vi "Set Clip Plane (no reference).vi"(8 "error in (no error)":errorcluster, 9 "Clip Plane State":enum16{"Inherit Value", "Off", "On"}(ring), 10 "Clip Plane Refnum In":refnum<vi>, 11 "Scene Object In":refnum<vi>) -> (0 "error out":errorcluster, 3 "Scene Object Out":refnum<vi>)   [LabVIEW 2017, in "NI_3D Picture Control.lvlib"]
doc: "Defines the plane beyond which LabVIEW clips, or does not render, surfaces in a scene."
uses:
  <vilib>/picture/3D Picture Control/NI_3D Picture Control.lvlib
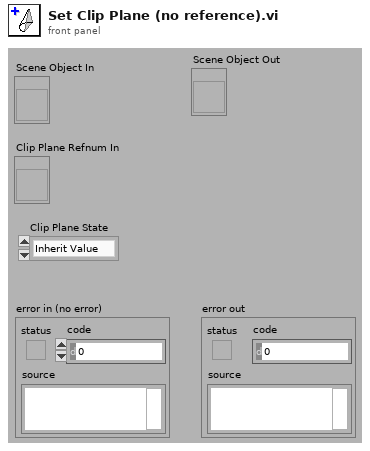
[diagram p1: front panel]
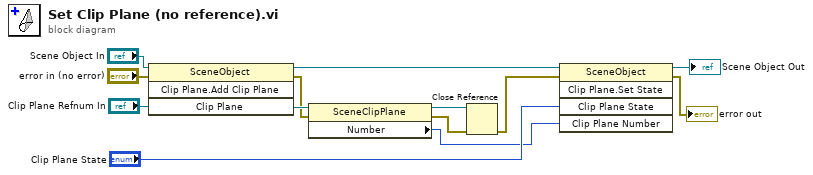
[diagram p0: block diagram]
diagram:
  n1 = invoke class="SceneObject" method="Clip Plane.Add Clip Plane"(reference="Scene Object In", error in="error in (no error)", "Clip Plane"="Clip Plane Refnum In") -> (reference out=w9:refnum<vi>, error out=w4:errorcluster, "Clip Plane"=w6:refnum<vi>)  [unwired: 1 in, 1 out]
  n2 = property class="SceneClipPlane"(reference=w6, error in=w4) -> (reference out=w3:refnum<vi>, error out=w2:errorcluster, "Number"=w5:i32)
  n3 = Close Reference(reference=w3, error in (no error)=w2) -> (error out=w1:errorcluster)
  n4 = invoke class="SceneObject" method="Clip Plane.Set State"(reference=w9, error in=w1, "Clip Plane State"="Clip Plane State", "Clip Plane Number"=w5) -> (reference out=→"Scene Object Out":refnum<vi>, error out=→"error out":errorcluster)  [unwired: 1 in, 3 out]
